vi "Driver Globals.vi"() -> ()   [LabVIEW 2019]
panel:
  in  "ReverseConveyor":bool
  out "VisionAligned?":bool
  in  "ZAxis":dbl
  in  "SwerveSpeed":dbl
  in  "StrafeAngle":dbl
  in  "Climb":bool
  in  "YawManual":dbl
  in  "Intake":bool
  in  "Cannon":bool
  in  "VisionAlign":bool
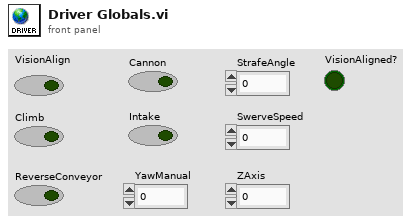
[diagram p1: front panel]
diagram:
